vi "RichToFlatniswitch_grpc_GetRelayPositionRequest.vi"(5 "OutputClusterType":T1, 11 "InputCluster":T3) -> (3 "OutputCluster":T1)   [LabVIEW 2021, in "NI Switch_client.lvlib"]
uses:
  NI Switch_client.lvlib
  niswitch_grpc_GetRelayPositionRequest.ctl
  nidevice_grpc_Session.ctl
  niswitch_grpc_GetRelayPositionRequest_Flat.ctl
  nidevice_grpc_Session_Flat.ctl
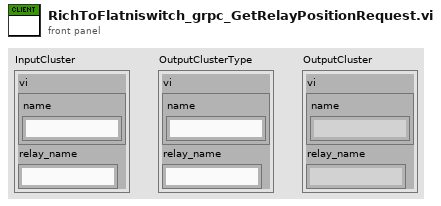
[diagram p1: front panel]
types:
  T1 = typedef "NI Switch_client.lvlib/niswitch_grpc_GetRelayPositionRequest_Flat.ctl" = cluster{"vi":T2, "relay_name":string}
  T2 = typedef "NI Switch_client.lvlib/nidevice_grpc_Session_Flat.ctl" = cluster{"name":string}
  T3 = typedef "NI Switch_client.lvlib/niswitch_grpc_GetRelayPositionRequest.ctl" = cluster{"vi":T4, "relay_name":string}
  T4 = typedef "NI Switch_client.lvlib/nidevice_grpc_Session.ctl" = cluster{"name":string}
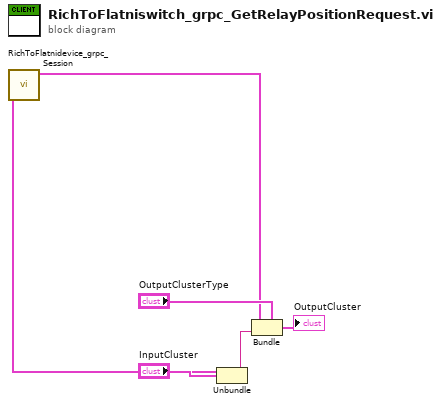
[diagram p0: block diagram]
diagram:
  n1 = Unbundle "Unbundle"("InputCluster") -> ("vi"=w3:T4, "relay_name"=w1:string)
  n2 = call "RichToFlatnidevice_grpc_Session.vi"("InputCluster"=w3) -> ("OutputCluster"=w2:T2)  [unwired: 10 in]
  n3 = Bundle "Bundle"(cluster="OutputClusterType", "vi"=w2, "relay_name"=w1) -> (→"OutputCluster":T1)
